vi "BlankControls_VI.vi"   [LabVIEW 2010]
uses:
  <vilib>/NXT/Dual Mode Library/Motors/MotorOn.vi
  <vilib>/NXT/Dual Mode Library/Sensors/Touch_Pressed.vi
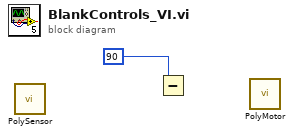
[diagram p0: block diagram]
diagram:
  n1 = call-poly <vilib>:"PolySensor.vi"() -> ()  [unwired: 3 in, 2 out]
  n2 = Subtract(x=90) -> ()  [unwired: 1 in, 1 out]
  n3 = call-poly <vilib>:"PolyMotor.vi"() -> ()  [unwired: 4 in, 1 out]
